vi "CRYSet Serial No Front Panel.vi"(11 "Vi Ref":refnum<vi>) -> ()   [LabVIEW 2013]
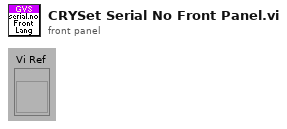
[diagram p1: front panel]
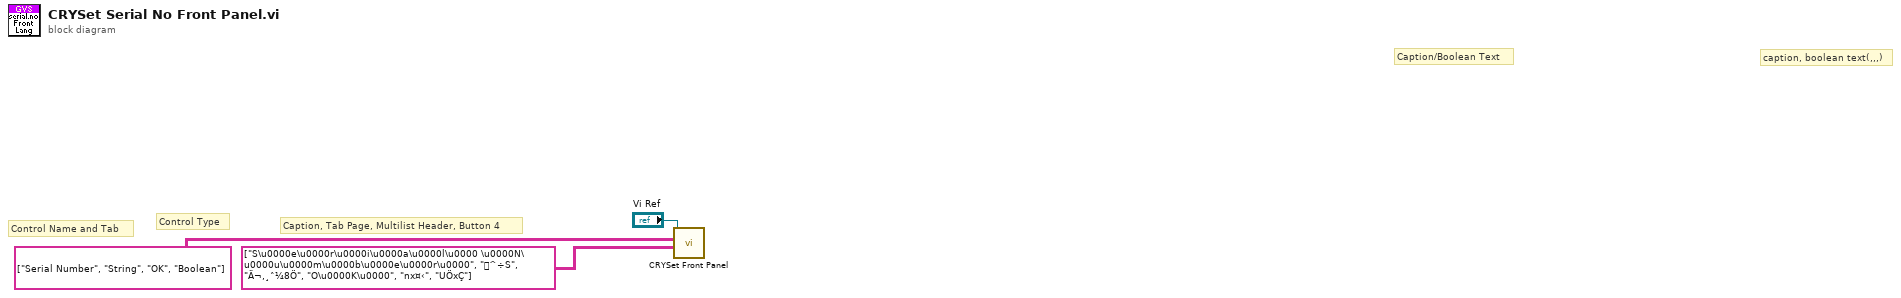
[diagram p0: block diagram]
diagram:
  # "Caption, Tab Page, Multilist Header, Button 4"
  # "Control Type"
  # "Control Name and Tab"
  # "caption, boolean text(,,,)"
  # "Caption/Boolean Text"
  n1 = call "CRYSet Front Panel.vi"("Caption(Boolean Text)"=string[][] [["S\u0000e\u0000r\u0000i\u0000a\u0000l\u0000 \u0000N\u0000u\u0000m\u0000b\u0000e\u0000r\u0000", "^÷S", "Ä¬,¸ˆ¼8Ö"], ["O\u0000K\u0000", "nx¤‹", "UÖxÇ"]], "Control ID and Type(Label Name, Type)"=string[][] [["Serial Number", "String"], ["OK", "Boolean"]], "Vi Ref"="Vi Ref") -> ()  [unwired: 9 in]
